vi "TS AUTO-DETECT.vi"() -> ()   [LabVIEW 2015]
uses:
  <vilib>/Utility/inputDevices.llb/joystickAcquire.vi
  <vilib>/Utility/inputDevices.llb/closeJoystick.vi
panel:
  out "Boolean":bool
  out "Found??":bool
  out "Actual":i32
  out "Current":i32
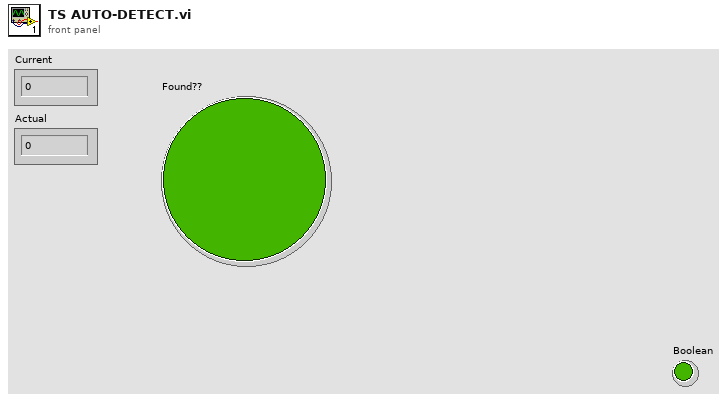
[diagram p1: front panel]
types:
  T1 = cluster{"button 1":bool, "button 2":bool, "button 3":bool, "button 4":bool, "button 5":bool, "button 6":bool, "button 7":bool, "button 8":bool, "button 9":bool, "button 10":bool, "button 11":bool, "button 12":bool, "button 13":bool, "button 14":bool, "button 15":bool, "button 16":bool, "button 17":bool, "button 18":bool, "button 19":bool, "button 20":bool, "button 21":bool, "button 22":bool, "button 23":bool, "button 24":bool, "button 25":bool, "button 26":bool, "button 27":bool, "button 28":bool, "button 29":bool, "button 30":bool, "button 31":bool, "button 32":bool}
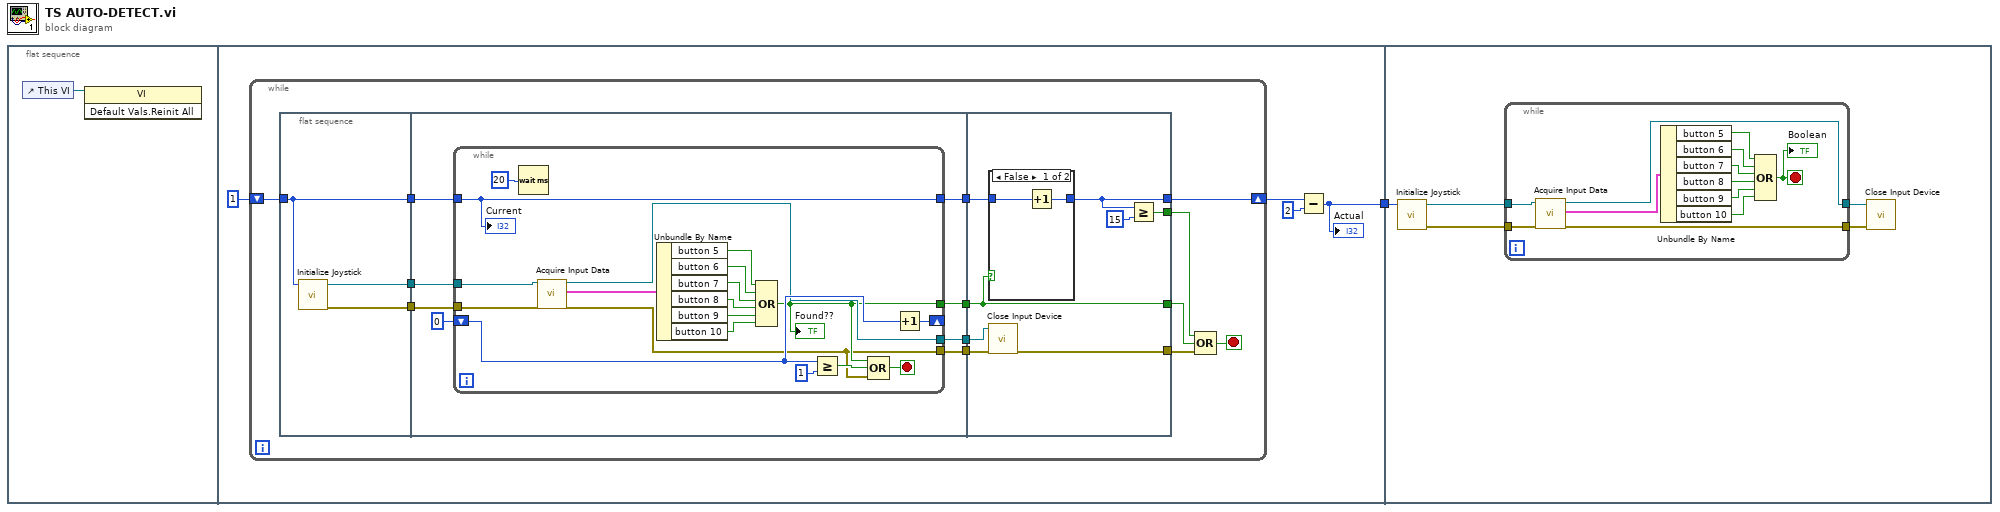
[diagram p0: block diagram]
diagram:
  n1 = flat-sequence {
    tunnel: [w3] -> w1
    tunnel: w1 -> [w61]
    frame #0 {
      n2 = control-ref of="This VI"() -> (w2:refnum<vi>)
      n3 = invoke class="VI" method="Default Vals.Reinit All"(reference=w2) -> ()  [unwired: 2 in, 3 out]
    }
    frame #1 {
      n4 = while {
        shift-right: [w8] -> w4
        shift-left: 1 -> [w13]
        stop <- w12 stop-if-true
        n5 = flat-sequence {
          tunnel: [w22] -> w19
          tunnel: [w21] -> w18
          tunnel: [w20] -> w14
          tunnel: w13 -> [w20]
          tunnel: w19 -> [w30]
          tunnel: w18 -> [w29]
          tunnel: [w27] -> w17
          tunnel: [w26] -> w16
          tunnel: [w25] -> w15
          tunnel: w14 -> [w24]
          tunnel: [w23] -> w10
          tunnel: w17 -> [w57]
          tunnel: w16 -> [w56]
          tunnel: w15 -> [w52]
          tunnel: [w54] -> w11
          tunnel: w10 -> [w53]
          tunnel: [w53] -> w9
          tunnel: [w51] -> w8
          tunnel: [w50] -> w7
          frame #0 {
            n6 = call <vilib>:"Initialize Joystick.vi"("device index"=w20) -> ("error out"=w21:errorcluster, "device ID"=w22:refnum<k1>)  [unwired: 9 in]
          }
          frame #1 {
            n7 = while {
              tunnel: w30 -> [w48]
              tunnel: w29 -> [w47]
              shift-right: [w39] -> _
              shift-left: 0 -> [w38]
              tunnel: [w34] -> w27
              tunnel: [w31] -> w26
              tunnel: [w33] -> w25
              tunnel: w24 -> [w33]
              tunnel: [w32] -> w23
              stop <- w35 stop-if-true
              n8 = Wait (ms)(milliseconds to wait=u32 20) -> ()  [unwired: 1 out]
              n9 = call-poly <vilib>:"Acquire Input Data.vi"("device ID"=w48, "error in (no error)"=w47) -> ("device ID"=w34:refnum<k1>, "button info"=w46:T1, "error out"=w31:errorcluster)  [unwired: 13 in, 2 out]
              n10 = Unbundle By Name(w46) -> ("button 5"=w45:bool, "button 6"=w44:bool, "button 7"=w43:bool, "button 8"=w42:bool, "button 9"=w41:bool, "button 10"=w40:bool)
              n11 = Compound Arithmetic op=OR(w45, w44, w43, w42, w41, w40) -> (w32:bool)
              "Found??" <- w32
              n12 = Greater Or Equal?(x=w38, y=1) -> (x >= y?=w36:bool)
              n13 = Compound Arithmetic op=OR(w32, w36, w31) -> (w35:bool)
              n14 = Increment(x=w38) -> (x+1=w39:i32)
              "Current" <- w33
            }
          }
          frame #2 {
            n15 = case shown="False" w53 {
              tunnel: w52 -> [w59 w60]
              tunnel: [w58 w60] -> w51
              frame False {
                n16 = Increment(x=w59) -> (x+1=w58:i32)
              }
              frame True {
              }
            }
            n17 = call-poly <vilib>:"Close Input Device.vi"("error in (no error)"=w56, "device ID"=w57) -> ("error out"=w50:errorcluster)  [unwired: 8 in]
            n18 = Greater Or Equal?(x=w51, y=15) -> (x >= y?=w54:bool)
          }
        }
        n19 = Compound Arithmetic op=OR(w11, w9, w7) -> (w12:bool)
      }
      n20 = Subtract(x=w4, y=2) -> (x-y=w3:i32)
      "Actual" <- w3
    }
    frame #2 {
      n21 = call <vilib>:"Initialize Joystick.vi"("device index"=w61) -> ("error out"=w64:errorcluster, "device ID"=w65:refnum<k1>)  [unwired: 9 in]
      n22 = while {
        tunnel: w65 -> [w77]
        tunnel: w64 -> [w76]
        tunnel: [w67] -> w63
        tunnel: [w66] -> w62
        stop <- w68 stop-if-true
        n23 = call-poly <vilib>:"Acquire Input Data.vi"("device ID"=w77, "error in (no error)"=w76) -> ("device ID"=w67:refnum<k1>, "button info"=w75:T1, "error out"=w66:errorcluster)  [unwired: 13 in, 2 out]
        n24 = Unbundle By Name(w75) -> ("button 5"=w74:bool, "button 6"=w73:bool, "button 7"=w72:bool, "button 8"=w71:bool, "button 9"=w70:bool, "button 10"=w69:bool)
        n25 = Compound Arithmetic op=OR(w74, w73, w72, w71, w70, w69) -> (w68:bool)
        "Boolean" <- w68
      }
      n26 = call-poly <vilib>:"Close Input Device.vi"("error in (no error)"=w62, "device ID"=w63) -> ()  [unwired: 8 in, 1 out]
    }
  }
